vi "Standartabweichung.vi"(8 "Breite":i32=60, 11 "wave":cluster{"x":dbl[], "y":dbl[]} {"x" format="%<%H:%M:%S%3u %d/%m/%Y>T"; "y" format="%#_14f"}) -> (1 "residue":dbl format="%_6g", 3 "Graph_sdv":cluster{"X":dbl[], "Y":dbl[]}(graph))   [LabVIEW 2010, in "Licor-Steuerung.lvlib"]
uses:
  Licor-Steuerung.lvlib
  <vilib>/Analysis/NI_AALBase.lvlib
panel:
  out "Array 2":i32[](array[numeric])
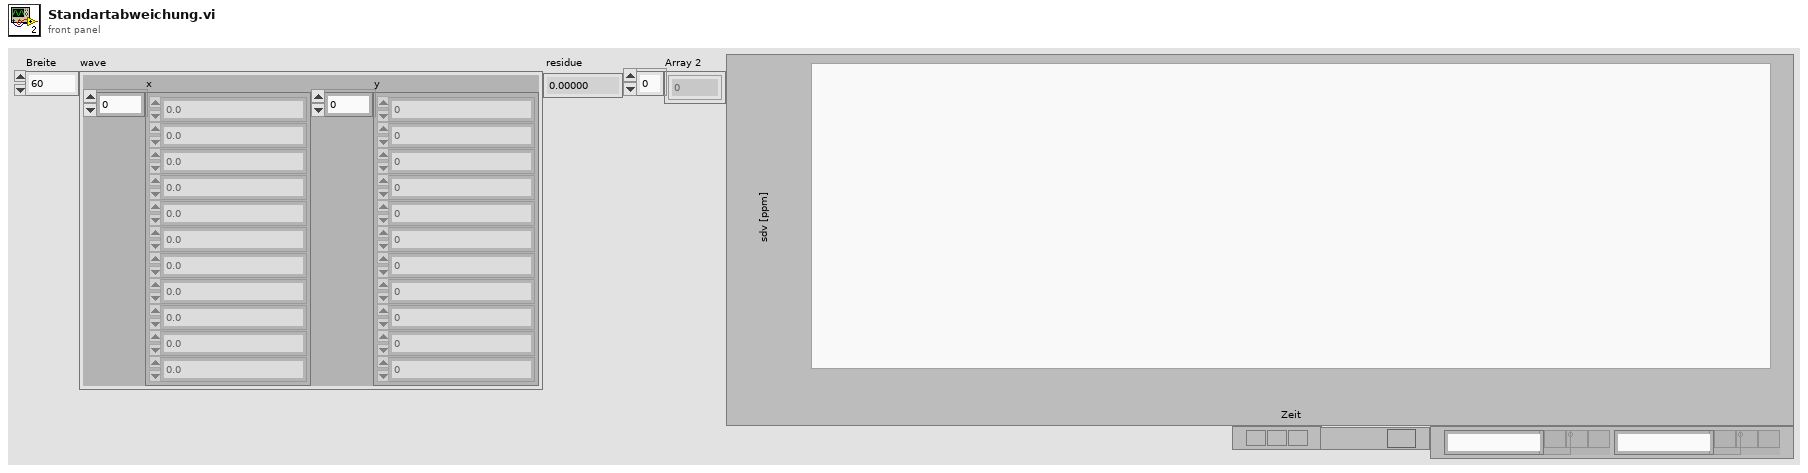
[diagram p1: front panel]
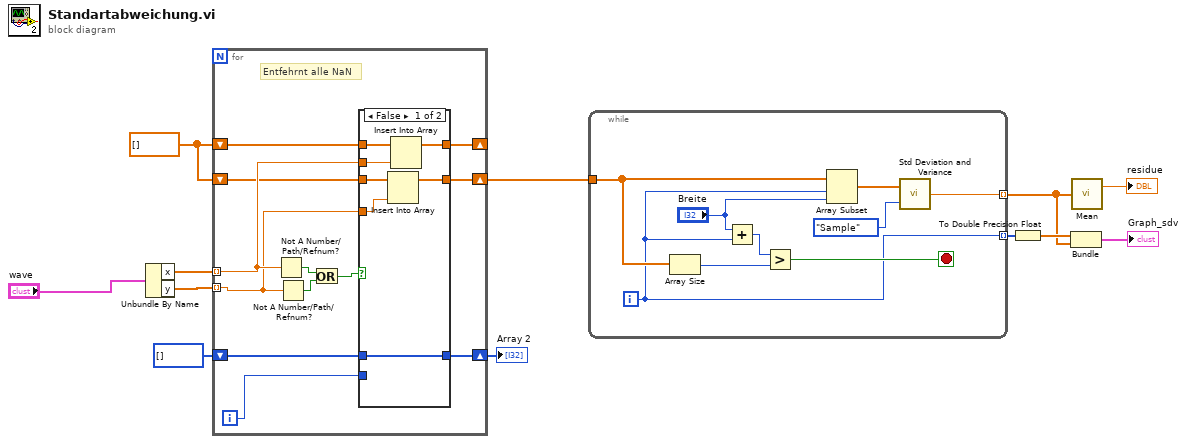
[diagram p0: block diagram]
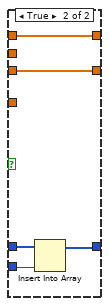
[diagram p2: hidden frame]
diagram:
  w10 = dbl[] []
  n1 = Unbundle By Name("wave") -> ("x"=w12:dbl[], "y"=w11:dbl[])
  n2 = for {
    tunnel: w12 -> [w22] mode=indexing
    tunnel: w11 -> [w21] mode=indexing
    shift-right: [w20] -> _
    shift-left: w10 -> [w18]
    shift-right: [w19] -> w6
    shift-left: w10 -> [w17]
    shift-right: [w14] -> w8
    shift-left: i32[] [] -> [w13]
    i -> [w15]
    # "Entfehrnt alle NaN"
    n3 = Not A Number/Path/Refnum?(number/path/refnum=w22) -> (NaN/Path/Refnum?=w24:bool)
    n4 = Not A Number/Path/Refnum?(number/path/refnum=w21) -> (NaN/Path/Refnum?=w23:bool)
    n5 = Or(x=w24, y=w23) -> (x .or. y?=w16:bool)
    n6 = case shown="False" w16 {
      tunnel: w22 -> [w31 _]
      tunnel: w21 -> [w30 _]
      tunnel: [w29 w36] -> w20
      tunnel: [w28 w35] -> w19
      tunnel: w18 -> [w27 w36]
      tunnel: w17 -> [w26 w35]
      tunnel: w15 -> [_ w33]
      tunnel: [w25 w32] -> w14
      tunnel: w13 -> [w25 w34]
      frame False {
        n7 = Insert Into Array(array=w26, new element=w30) -> (w28:dbl[])  [unwired: 1 in]
        n8 = Insert Into Array(array=w27, new element=w31) -> (w29:dbl[])  [unwired: 1 in]
      }
      frame True {
        n9 = Insert Into Array(array=w34, new element=w33) -> (w32:i32[])  [unwired: 1 in]
      }
    }
  }
  "Array 2" <- w8
  n10 = while {
    tunnel: w6 -> [w42]
    tunnel: [w43] -> w3 mode=indexing
    tunnel: [w37] -> w5 mode=indexing
    i -> [w37]
    stop <- w38 stop-if-true
    n11 = Array Size(array=w42) -> (size(s)=w39:i32)
    n12 = Add(x="Breite", y=w37) -> (x+y=w40:i32)
    n13 = Greater?(x=w40, y=w39) -> (0:w38:bool)
    n14 = Array Subset(array=w42, index=w37, length="Breite") -> (w45:dbl[])
    n15 = call <vilib>:"Std Deviation and Variance.vi"("X"=w45, "Weighting (Sample)"=enum16{"Sample", "Population"}."Sample") -> ("standard deviation"=w43:dbl)  [unwired: 2 out]
  }
  n16 = To Double Precision Float(number=w5) -> (double precision float=w4:dbl[])
  n17 = Bundle(w4, w3) -> (→"Graph_sdv":cluster{dbl[], dbl[]})  [unwired: 1 in]
  n18 = call <vilib>:"Mean.vi"("X"=w3) -> ("mean"=→"residue":dbl)  [unwired: 1 out]
